vi "linie_mit_pfeil.vi"(4 "Richtungspfeillänge":sgl, 6 "Angle":sgl, 7 "Color":u32, 8 "Boolean":bool, 9 "x":sgl, 10 "y":sgl, 11 "Refnum in":T1) -> (3 "Refnum out":T1)   [LabVIEW 2014]
uses:
  <vilib>/vision/Image Controls.llb/IMAQ Image.ctl
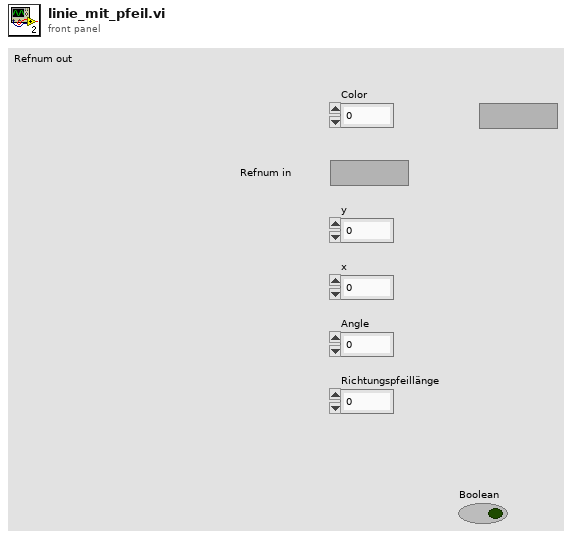
[diagram p1: front panel]
types:
  T1 = typedef "IMAQ Image.ctl" = refnum<image>
  T2 = cluster{"[0]":cluster{"x":sgl, "y":sgl}, "[1]":cluster{"x":sgl, "y":sgl}, "[2]":cluster{"x":sgl, "y":sgl}, "[3]":cluster{"x":sgl, "y":sgl}, "[4]":cluster{"x":sgl, "y":sgl}, "[5]":cluster{"x":sgl, "y":sgl}, "[6]":cluster{"x":sgl, "y":sgl}, "[7]":cluster{"x":sgl, "y":sgl}, "[8]":cluster{"x":sgl, "y":sgl}}
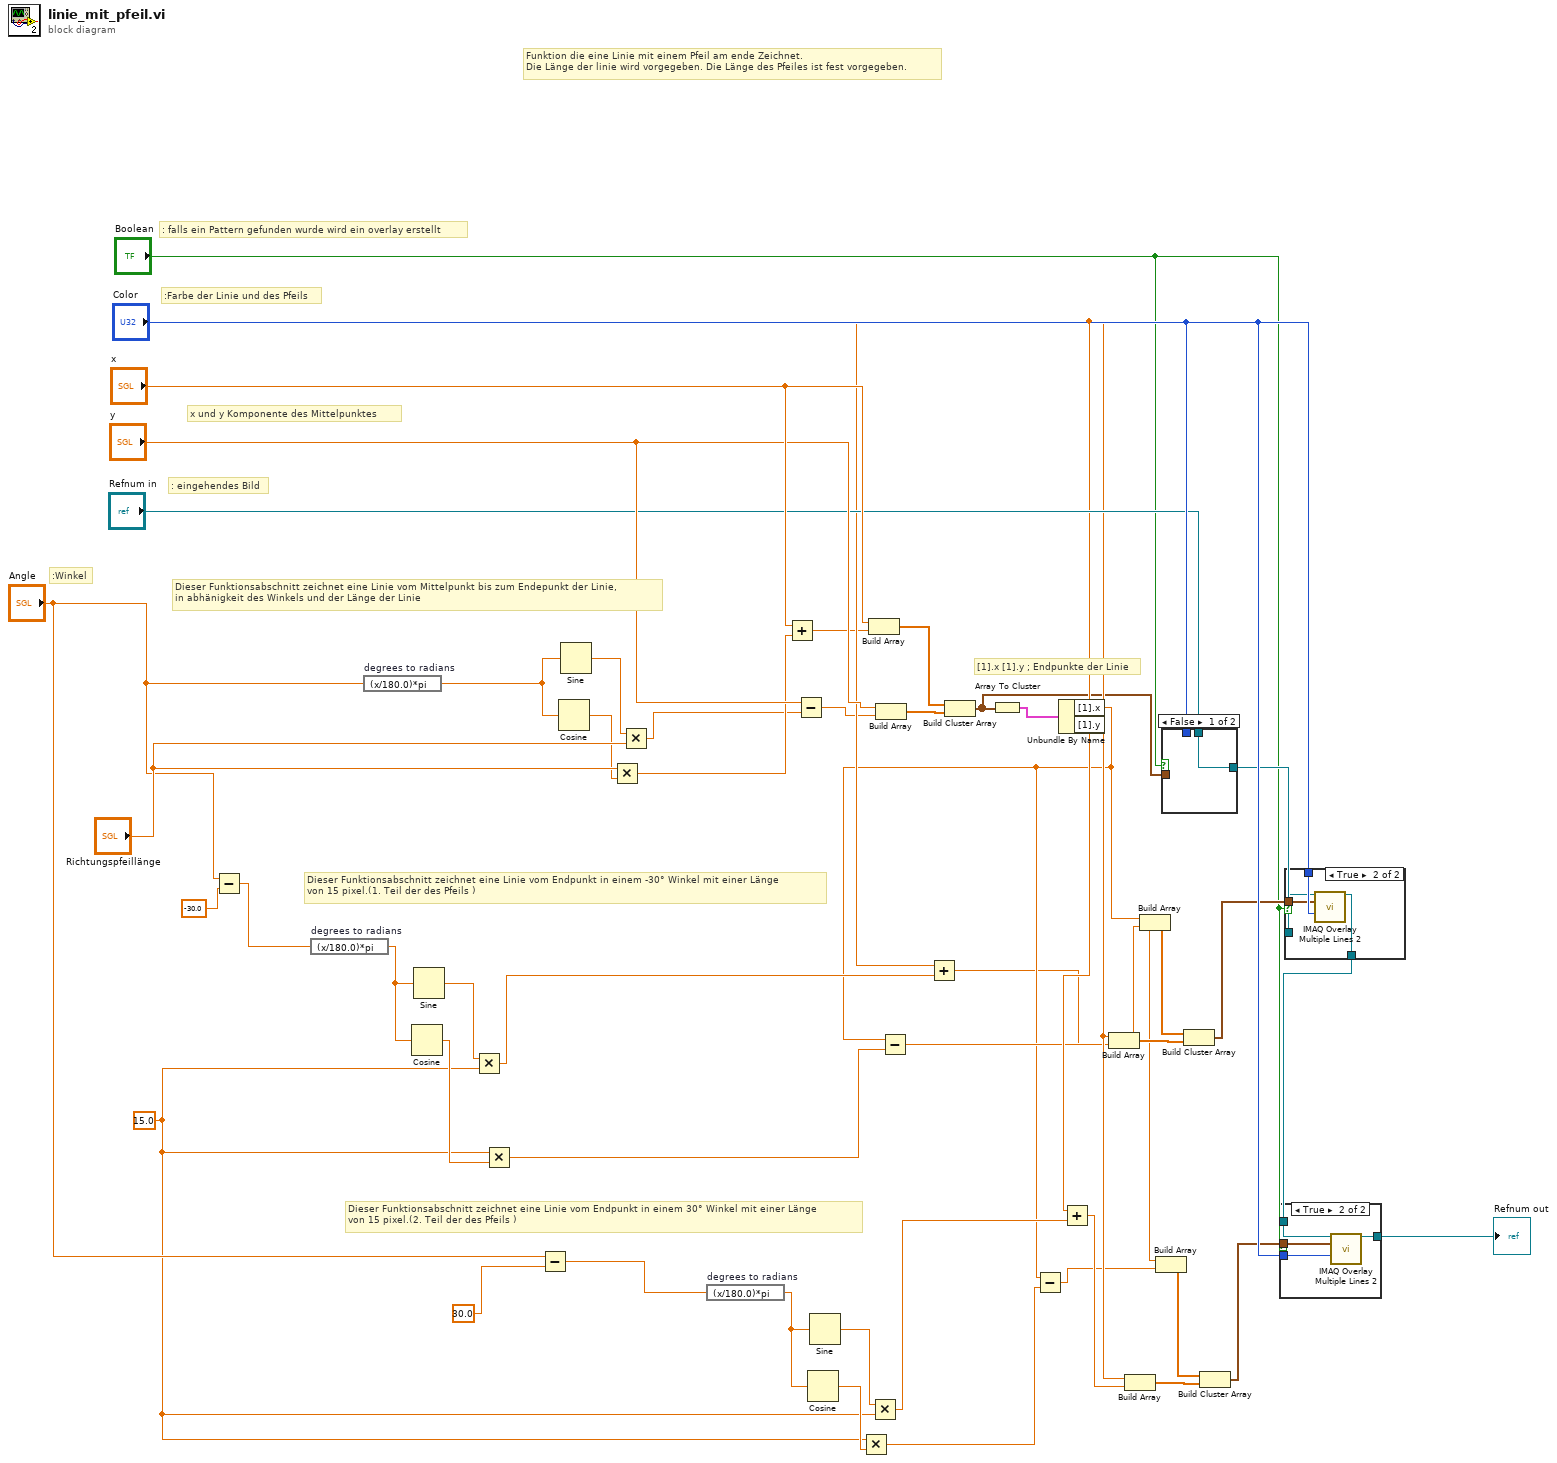
[diagram p0: block diagram]
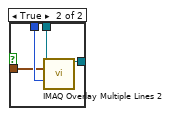
[diagram p4: hidden frame]
diagram:
  w4 = sgl 15.0 ("y")
  # "Dieser Funktionsabschnitt zeichnet eine Linie vom Endpunkt in einem 30° Winkel mit einer Länge \nvon 15 pixel.(2. Teil der des Pfeils )"
  # "Dieser Funktionsabschnitt zeichnet eine Linie vom Endpunkt in einem -30° Winkel mit einer Länge \nvon 15 pixel.(1. Teil der des Pfeils )"
  # "[1].x [1].y ; Endpunkte der Linie"
  # "Dieser Funktionsabschnitt zeichnet eine Linie vom Mittelpunkt bis zum Endepunkt der Linie, \nin abhänigkeit des Winkels und der Länge der Linie"
  # ":Winkel"
  # ": eingehendes Bild"
  # "x und y Komponente des Mittelpunktes"
  # ":Farbe der Linie und des Pfeils"
  # ": falls ein Pattern gefunden wurde wird ein overlay erstellt"
  # "Funktion die eine Linie mit einem Pfeil am ende Zeichnet.\nDie Länge der linie wird vorgegeben. Die Länge des Pfeiles ist fest vorgegeben."
  n1 = Subtract(x="Angle", y=sgl -30.0) -> (x-y=w22:sgl)
  n2 = expression code="(x/180.0)*pi" "degrees to radians"(w22) -> (w19:sgl)
  n3 = expression code="(x/180.0)*pi" "degrees to radians"("Angle") -> (w11:sgl)
  n4 = Cosine(x=w19) -> (cos(x)=w20:sgl)
  n5 = Sine(x=w19) -> (sin(x)=w21:sgl)
  n6 = Multiply(x=w21, y=w4) -> (x*y=w14:sgl)
  n7 = Multiply(x=w4, y=w20) -> (x*y=w15:sgl)
  n8 = Subtract(x="Angle", y=sgl 30.0) -> (x-y=w36:sgl)
  n9 = Cosine(x=w11) -> (cos(x)=w12:sgl)
  n10 = Sine(x=w11) -> (sin(x)=w13:sgl)
  n11 = Multiply(x="Richtungspfeillänge", y=w12) -> (x*y=w6:sgl)
  n12 = Multiply(x=w13, y="Richtungspfeillänge") -> (x*y=w5:sgl)
  n13 = expression code="(x/180.0)*pi" "degrees to radians"(w36) -> (w33:sgl)
  n14 = Add(x="x", y=w6) -> (x+y=w7:sgl)
  n15 = Subtract(x="y", y=w5) -> (x-y=w8:sgl)
  n16 = Cosine(x=w33) -> (cos(x)=w34:sgl)
  n17 = Sine(x=w33) -> (sin(x)=w35:sgl)
  n18 = Multiply(x=w4, y=w34) -> (x*y=w28:sgl)
  n19 = Build Array("x", w7) -> (w10:sgl[])
  n20 = Multiply(x=w35, y=w4) -> (x*y=w27:sgl)
  n21 = Build Array("y", w8) -> (w9:sgl[])
  n22 = Build Cluster Array(w10, w9) -> (w26:cluster{"x":sgl, "y":sgl}[])
  n23 = Array To Cluster(array=w26) -> (cluster=w24:T2)
  n24 = Unbundle By Name(w24) -> ("[1].x"=w3:sgl, "[1].y"=w38:sgl)
  n25 = Subtract(x=w3, y=w15) -> (x-y=w16:sgl)
  n26 = Add(x=w38, y=w14) -> (x+y=w2:sgl)
  n27 = Subtract(x=w3, y=w28) -> (x-y=w29:sgl)
  n28 = Add(x=w38, y=w27) -> (x+y=w30:sgl)
  n29 = Build Array(w38, w2) -> (w17:sgl[])
  n30 = Build Array(w38, w30) -> (w31:sgl[])
  n31 = Build Array(w3, w16) -> (w18:sgl[])
  n32 = Build Array(w3, w29) -> (w32:sgl[])
  n33 = case shown="False" "Boolean" {
    tunnel: "Color" -> [_ w53]
    tunnel: "Refnum in" -> [w49 w52]
    tunnel: w26 -> [_ w51]
    tunnel: [w49 w50] -> w25
    frame False {
    }
    frame True {
      n34 = call "IMAQ Overlay Multiple Lines 2"("Image"=w52, "Line End Points"=w51, "Color"=w53) -> ("Image Out"=w50:T1)  [unwired: 11 in, 1 out]
    }
  }
  n35 = Build Cluster Array(w18, w17) -> (w23:cluster{"x":sgl, "y":sgl}[])
  n36 = Build Cluster Array(w32, w31) -> (w37:cluster{"x":sgl, "y":sgl}[])
  n37 = case shown="True" "Boolean" {
    tunnel: "Color" -> [_ w58]
    tunnel: [w54 w57] -> w39
    tunnel: w25 -> [w54 w56]
    tunnel: w23 -> [_ w55]
    frame False {
    }
    frame True {
      n38 = call "IMAQ Overlay Multiple Lines 2"("Image"=w56, "Line End Points"=w55, "Color"=w58) -> ("Image Out"=w57:T1)  [unwired: 11 in, 1 out]
    }
  }
  n39 = case shown="True" "Boolean" {
    tunnel: "Color" -> [_ w63]
    tunnel: [w59 w62] -> w43
    tunnel: w39 -> [w59 w61]
    tunnel: w37 -> [_ w60]
    frame False {
    }
    frame True {
      n40 = call "IMAQ Overlay Multiple Lines 2"("Image"=w61, "Line End Points"=w60, "Color"=w63) -> ("Image Out"=w62:T1)  [unwired: 11 in, 1 out]
    }
  }
  "Refnum out" <- w43
